vi "ORS_WW-LinearizeFFTLineArray.vi"(0 "Ch1 Michelson":dbl[][](array[numeric]), 1 "DLL path":path=path "c:/", 2 "Linearization method":u16, 4 "RecalFringePhaseFit":dbl[](array[numeric]), 5 "RecalFringePhaseFit inverted":dbl[](array[numeric]) caption="inverted Hilbert in", 6 "Linearizer: Interpol. method":i32, 7 "Use DLL":bool, 11 "Window parameter":dbl=nan, 13 "Window":T1 items=["Rectangle"=0, "Hanning"=1, "Hamming"=2, "Blackman-Harris"=3, "Exact Blackman"=4, "Blackman"=5, "Flat Top"=6, "4 Term B-Harris "=7, "7 Term B-Harris"=8, "Low Sidelobe"=9, "Blackman Nuttall"=11, "Triangle"=30, "Bartlett-Hanning"=31, "Bohman"=32, "Parzen"=33, "Welch"=34, "Kaiser"=60, "Dolph-Chebyshev"=61, "Gaussian"=62], 17 "# zeros added":i32) -> (14 "Output":dbl[][](array[numeric]), 15 "error count":i32)   [LabVIEW 2014]
uses:
  <vilib>/Analysis/4window.llb/windowTd.ctl
  <vilib>/Analysis/2dsp.llb/Real FFT.vi
  <vilib>/Analysis/4window.llb/Symmetric Window (DBL).vi
  <vilib>/Analysis/2dsp.llb/Zero Padder (DBL).vi
  <vilib>/Analysis/NI_AALPro.lvlib
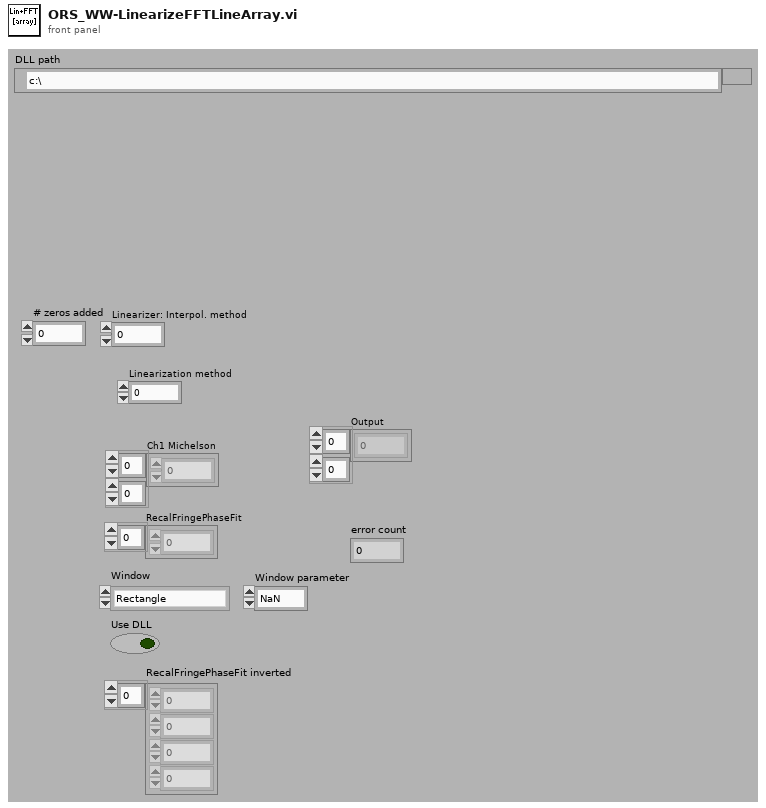
[diagram p1: front panel]
types:
  T1 = typedef "NI_AALPro.lvlib/windowTd.ctl" = u32
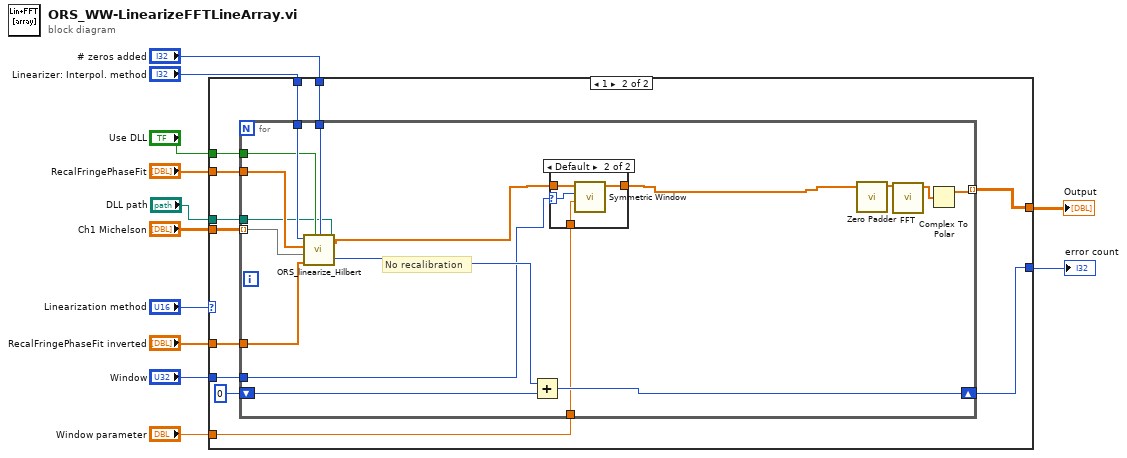
[diagram p0: block diagram]
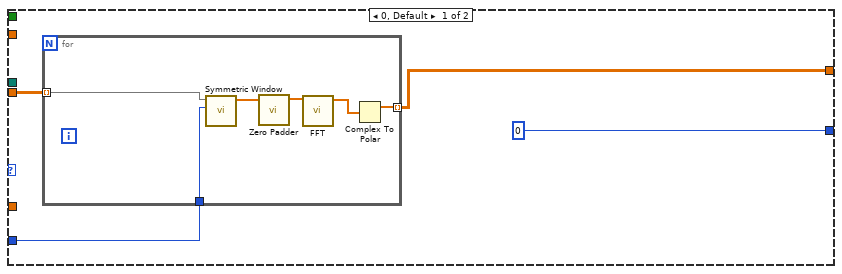
[diagram p2: hidden frame]
diagram:
  n1 = case shown="1" "Linearization method" {
    tunnel: "Ch1 Michelson" -> [w15 w31]
    tunnel: "Window" -> [w16 w27]
    tunnel: [0 w33] -> w10
    tunnel: "RecalFringePhaseFit inverted" -> [_ w32]
    tunnel: "RecalFringePhaseFit" -> [_ w30]
    tunnel: "Use DLL" -> [_ w29]
    tunnel: "Linearizer: Interpol. method" -> [_ w28]
    tunnel: [w14 w26] -> w4
    tunnel: "Window parameter" -> [_ w25]
    tunnel: "# zeros added" -> [_ w24]
    tunnel: "DLL path" -> [_ w23]
    frame 0, Default {
      n2 = for {
        tunnel: [w20] -> w14 mode=indexing
        tunnel: w16 -> [w18]
        tunnel: w15 -> [w17] mode=indexing
        n3 = call-poly <vilib>:"Symmetric Window.vi"("window"=w18, "X"=w17) -> ("Windowed X"=w19:dbl[])  [unwired: 8 in, 1 out]
        n4 = call-poly <vilib>:"Zero Padder.vi"("Input Array"=w19) -> ("Zero Padded Array"=w22:dbl[])  [unwired: 10 in]
        n5 = call-poly <vilib>:"FFT.vi"("X"=w22) -> ("FFT {X}"=w21:cdb[])  [unwired: 9 in, 1 out]
        n6 = Complex To Polar(r * e^(i*theta)=w21) -> (r=w20:dbl[])  [unwired: 1 out]
      }
    }
    frame 1 {
      # "No recalibration"
      n7 = for {
        tunnel: [w49] -> w26 mode=indexing
        shift-right: [w48] -> w33
        shift-left: 0 -> [w47]
        tunnel: w32 -> [w43]
        tunnel: w31 -> [w45] mode=indexing
        tunnel: w30 -> [w44]
        tunnel: w29 -> [w42]
        tunnel: w28 -> [w46]
        tunnel: w27 -> [w39]
        tunnel: w25 -> [w37]
        tunnel: w24 -> [w36]
        tunnel: w23 -> [w35]
        n8 = call "ORS_linearize_Hilbert.vi"("DLL path"=w35, "Use DLL"=w42, "# zeros added"=w36, "inverted Hilbert in"=w43, "Ch1 Michelson"=w45, "Hilbert in"=w44, "interpolation method"=w46) -> ("error count"=w41:i32, "Ch1 linearized"=w40:dbl[])  [unwired: 3 in]
        n9 = Add(x=w41, y=w47) -> (x+y=w48:i32)
        n10 = case shown="Default" w39 {
          selector: w39 -> [_ w54]
          tunnel: [w52 w56] -> w38
          tunnel: w40 -> [w52 w55]
          tunnel: w37 -> [_ w53]
          frame 0 {
          }
          frame Default {
            n11 = call-poly <vilib>:"Symmetric Window.vi"("window parameter"=w53, "window"=w54, "X"=w55) -> ("Windowed X"=w56:dbl[])  [unwired: 7 in, 1 out]
          }
        }
        n12 = call-poly <vilib>:"Zero Padder.vi"("Input Array"=w38) -> ("Zero Padded Array"=w51:dbl[])  [unwired: 10 in]
        n13 = call-poly <vilib>:"FFT.vi"("X"=w51) -> ("FFT {X}"=w50:cdb[])  [unwired: 9 in, 1 out]
        n14 = Complex To Polar(r * e^(i*theta)=w50) -> (r=w49:dbl[])  [unwired: 1 out]
      }
    }
  }
  "Output" <- w4
  "error count" <- w10
